vi "Actor Core.vi"(8 "error in":errorcluster, 11 "Fluke 2625A (Hydra II) in":refnum<class "Fluke 2625A (Hydra II).lvclass">) -> (0 "error out 2":errorcluster, 3 "Actor out":refnum<class "Actor.lvclass">)   [LabVIEW 2013, in "Generic Data Logger.lvlib" / "Fluke 2625A (Hydra II).lvlib" / "Fluke 2625A (Hydra II).lvclass"]
doc: "(<B>Filename</B>: Actor Framework.lvlib:Actor.lvclass:Actor Core.vi)\n\nReceives messages to the actor, reacts to them, and initiates any error handling that may shut the actor down.\n\nDescendant classes may override this VI to append parallel tasks for the actor to complete while it handles messages. Overrides use the Call Parent Method node."
uses:
  Fluke 2625A (Hydra II).lvclass
  <vilib>/ActorFramework/Actor/Actor.lvclass
  Generic Data Logger Card Class/Generic Data Logger Card.lvclass
  Generic Instrument/Generic Card/Generic Card.lvclass/Generic Card.ctl
  Generic Data Logger Card Class/Generic Data Logger Card.lvclass/Generic Data Logger Card.ctl
  Generic Data Logger Class/Generic Data Logger.lvclass
  <vilib>/ActorFramework/Actor/Actor.lvclass/Actor.ctl
  <vilib>/ActorFramework/Message Enqueuer/Message Enqueuer.lvclass/Message Enqueuer.ctl
  <vilib>/ActorFramework/Stop Msg/Stop Msg.lvclass/Stop Msg.ctl
  <vilib>/ActorFramework/Message Enqueuer/Init from Existing Queue.vi
  <vilib>/ActorFramework/Message Enqueuer/Enqueue.vi
  <vilib>/ActorFramework/Message Enqueuer/Enqueue Critical.vi
  <vilib>/ActorFramework/Message Priority Queue/Priority Enqueue.vi
  <vilib>/ActorFramework/Message Enqueuer/Message Enqueuer.lvclass
  Generic Data Logger Messages/Measure Msg/Measure Msg.lvclass
  <vilib>/ActorFramework/Stop Msg/Stop Msg.lvclass
  Generic Instrument/Generic Card/Generic Card.lvclass
panel:
  in  "Generic Data Logger Card in":refnum<class "Generic Data Logger Card.lvclass">
  out "Array of Channels":bool[](array[boolean])
  in  "Data Array":dbl[](array[numeric])
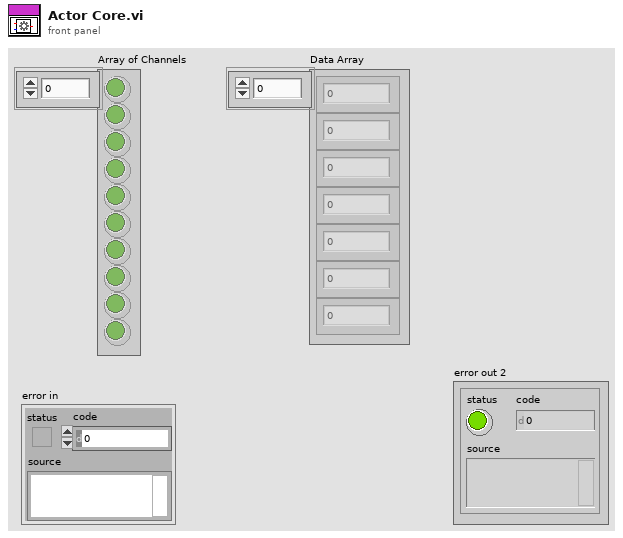
[diagram p1: front panel]
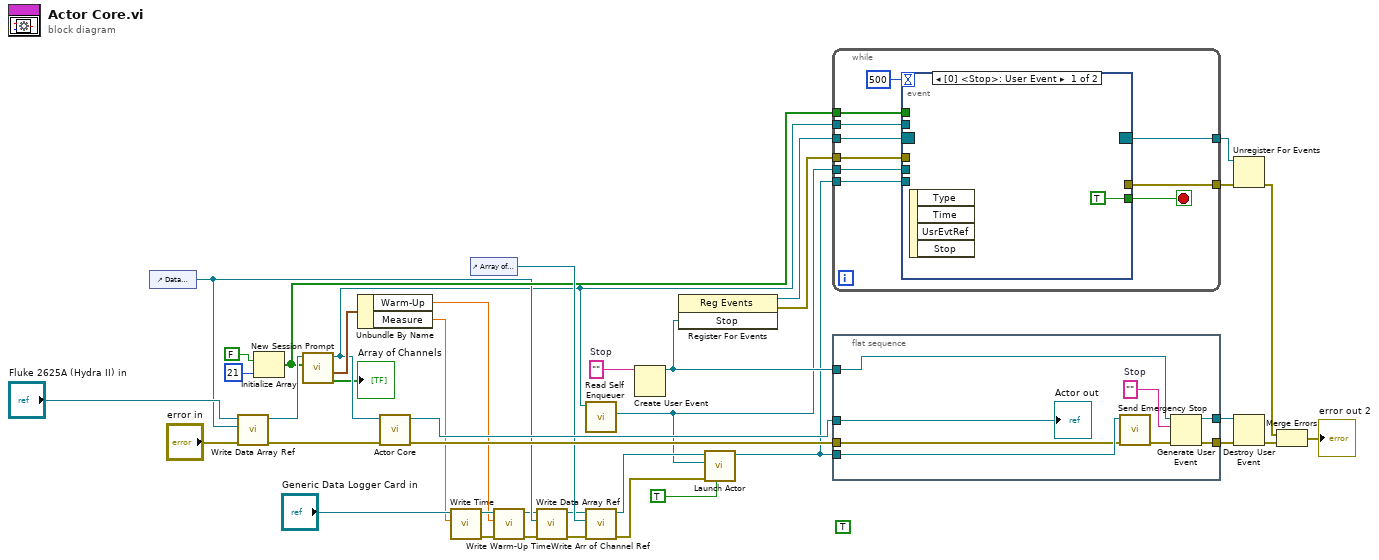
[diagram p0: block diagram]
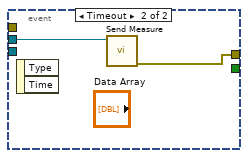
[diagram p2: hidden frame]
diagram:
  (unwired) TRUE ("Start/Stop")
  w36 = ""  # Stop
  n1 = control-ref of="Data Array"() -> (w12:refnum<vi>)
  n2 = call-dynamic "Write Data Array Ref.vi"("error in (no error)"="error in", "Data Array Ref"=w12, "Generic Instrument in"="Fluke 2625A (Hydra II) in") -> ("error out"=w2:errorcluster, "Generic Instrument out"=w16:refnum<class "Fluke 2625A (Hydra II).lvclass">)  [unwired: 7 in]
  n3 = Initialize Array(FALSE, 21 ("dimension size")) -> (w15:bool[])
  n4 = call "New Session Prompt.vi"("Array of channels in"=w15, "Generic Data Logger.lvlib:Fluke 2625A (Hydra II).lvlib:Fluke 2625A (Hydra II).lvclass"=w16) -> ("Array of channels out"=→"Array of Channels":bool[], "Time Cluster"=w6:cluster{"Warm-Up":dbl, "Measure":dbl}, "Generic Instrument out"=w3:refnum<class "Fluke 2625A (Hydra II).lvclass">)  [unwired: 7 in]
  n5 = Unbundle By Name(w6) -> ("Warm-Up"=w5:dbl, "Measure"=w4:dbl)
  n6 = call-parent "Actor Core.vi"("error in"=w2, "Actor in"=w3) -> ("error out"=w39:errorcluster, "Actor out"=w38:refnum<class "Actor.lvclass">)  [unwired: 8 in]
  n7 = call "Write Time .vi"("Time"=w4, "Generic Card in"="Generic Data Logger Card in") -> ("error out"=w7:errorcluster, "Generic Card out"=w11:refnum<class "Generic Data Logger Card.lvclass">)  [unwired: 8 in]
  n8 = control-ref of="Array of Channels"() -> (w30:refnum<vi>)
  n9 = call "Write Warm-Up Time.vi"("error in (no error)"=w7, "Warm-Up Time"=w5, "Generic Card in"=w11) -> ("error out"=w8:errorcluster, "Generic Card out"=w9:refnum<class "Generic Data Logger Card.lvclass">)  [unwired: 7 in]
  n10 = call "Write Data Array Ref.vi"("error in (no error)"=w8, "Data Array Ref"=w12, "Generic Card in"=w9) -> ("error out"=w13:errorcluster, "Generic Card out"=w14:refnum<class "Generic Data Logger Card.lvclass">)  [unwired: 7 in]
  n11 = call <vilib>:"Read Self Enqueuer.vi"("Actor"=w3) -> ("Self Enqueuer"=w23:refnum<class "Message Enqueuer.lvclass">)  [unwired: 10 in]
  n12 = call "Write Arr of Channel Ref.vi"("error in (no error)"=w13, "Arr of Channel Ref"=w30, "Generic Data Logger Card in"=w14) -> ("error out"=w27:errorcluster, "Generic Data Logger Card out"=w29:refnum<class "Generic Data Logger Card.lvclass">)  [unwired: 7 in]
  n13 = Create User Event(user event datatype=w36) -> (user event=w35:refnum<user-event>)  [unwired: 1 in, 1 out]
  n14 = register-events(w35) -> (reference out=w24:refnum<event-registration>, error out=w20:errorcluster)  [unwired: 2 in]
  n15 = call <vilib>:"Launch Actor.vi"("Open Actor Core front panel? (F)"=TRUE, "error in (no error)"=w27, "Actor-to-Caller Enqueuer"=w23, "Actor"=w29) -> ("Caller-To-Actor Enqueuer"=w28:refnum<class "Message Enqueuer.lvclass">)  [unwired: 6 in, 1 out]
  n16 = while {
    tunnel: [w49] -> w25
    tunnel: w24 -> [w48]
    tunnel: w23 -> [w45]
    tunnel: w28 -> [w44]
    tunnel: w15 -> [w43]
    tunnel: w3 -> [w42]
    tunnel: w20 -> [w41]
    tunnel: [w40] -> w19
    stop <- w47 stop-if-true
    n17 = event shown="[0] <Stop>: User Event" {
      selector: w48 -> [_ _]
      dyn-events: [_ _] -> w49
      timeout: 500 -> [_ _]
      tunnel: [TRUE _] -> w47
      tunnel: w45 -> [_ w52]
      tunnel: w44 -> [_ _]
      tunnel: w43 -> [_ _]
      tunnel: w42 -> [_ _]
      tunnel: w41 -> [_ _]
      tunnel: [_ w51] -> w40
      event User Event {
        n18 = event-data() -> ()  [unwired: 1 in, 4 out]
      }
      event Timeout {
        n19 = event-data() -> ()  [unwired: 1 in, 2 out]
        n20 = call "Send Measure.vi"("Message Enqueuer"=w52) -> ("error out"=w51:errorcluster)  [unwired: 9 in, 1 out]
      }
    }
  }
  n21 = flat-sequence {
    tunnel: w39 -> [w54]
    tunnel: w38 -> [w60]
    tunnel: [w59] -> w37
    tunnel: w35 -> [w58]
    tunnel: [w57] -> w34
    tunnel: w28 -> [w55]
    frame #0 {
      w56 = ""  # Stop
      n22 = call <vilib>:"Send Emergency Stop.vi"("error in (no error)"=w54, "Message Enqueuer"=w55) -> ("error out"=w53:errorcluster)  [unwired: 9 in]
      n23 = Generate User Event(user event=w58, event data cluster=w56, error in=w53) -> (user event out=w59:refnum<user-event>, error out=w57:errorcluster)  [unwired: 1 in]
      "Actor out" <- w60
    }
  }
  n24 = Unregister For Events(event registration refnum=w25, error in=w19) -> (error out=w21:errorcluster)
  n25 = Destroy User Event(user event=w37, error in=w34) -> (error out=w17:errorcluster)
  n26 = Merge Errors(w21, w17) -> (→"error out 2":errorcluster)
